vi "1A_Calculate Temperature.vi"(3 "Therm_Offset":i32, 4 "Therm_Input":i32, 5 "Therm_Bias":i32, 6 "Temperature Data":string) -> (0 "RTherm":dbl, 1 "Temperature":dbl)   [LabVIEW 2010]
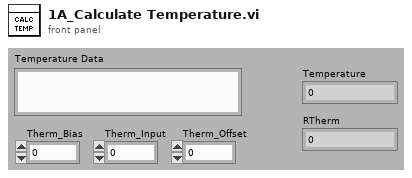
[diagram p1: front panel]
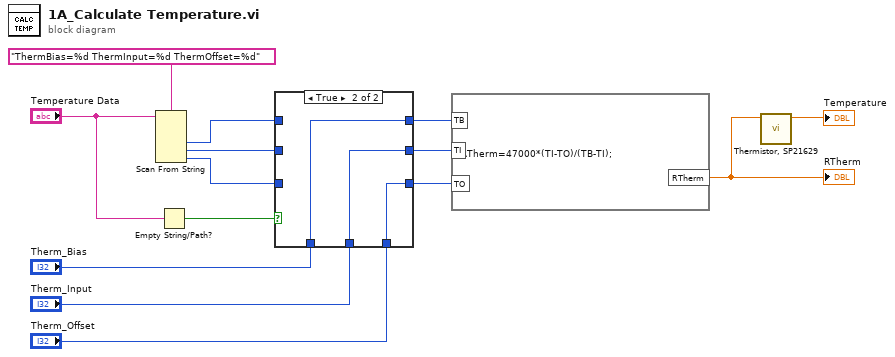
[diagram p0: block diagram]
diagram:
  n1 = Scan From String(format string="ThermBias=%d ThermInput=%d ThermOffset=%d", input string="Temperature Data") -> (output 1=w11:i32, output 2=w10:i32, output 3=w9:i32)  [unwired: 5 in, 3 out]
  n2 = Empty String/Path?(string/path="Temperature Data") -> (empty?=w12:bool)
  n3 = case shown="True" w12 {
    tunnel: w11 -> [w17 _]
    tunnel: w10 -> [w16 _]
    tunnel: w9 -> [w15 _]
    tunnel: [w17 w18] -> w8
    tunnel: [w16 w19] -> w7
    tunnel: [w15 w20] -> w6
    tunnel: "Therm_Offset" -> [_ w20]
    tunnel: "Therm_Input" -> [_ w19]
    tunnel: "Therm_Bias" -> [_ w18]
    frame False {
    }
    frame True {
    }
  }
  n4 = formula code="RTherm=47000*(TI-TO)/(TB-TI);"("TB"=w8, "TI"=w7, "TO"=w6) -> ("RTherm"=w2:dbl)
  "RTherm" <- w2
  n5 = call "Thermistor, SP21629.vi"("resistance (ohms)"=w2) -> ("temperature (C)"=→"Temperature":dbl)  [unwired: 9 in, 1 out]
